vi "Chroma 1905x Series Check Equipment.vi"(8 "error in (no error)":errorcluster, 11 "inst handle in":refnum<visa-resource-name>) -> (0 "error out":errorcluster, 2 "Equipment Error":bool, 3 "inst handle out":refnum<visa-resource-name>)   [LabVIEW 2025]
doc: "Contact Chroma\nTEL: +886-2-2298-3855 \nTEL: +886-3-397-5788 \nFAX: +886-2-2298-3596\nFAX: +886-3-327-4703 \nURL: http://www.chromaate.com \nE-mail: chroma@chroma.com.tw"
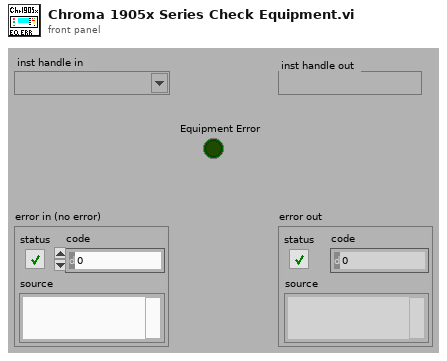
[diagram p1: front panel]
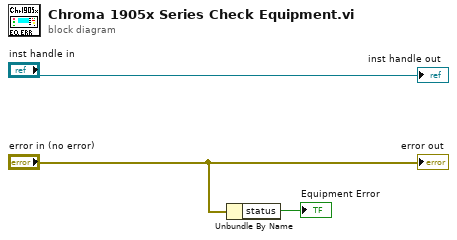
[diagram p0: block diagram]
diagram:
  n1 = Unbundle By Name("error in (no error)") -> ("status"=→"Equipment Error":bool)
  "inst handle out" <- "inst handle in"
  "error out" <- "error in (no error)"
